vi "Start.vi"(8 "error in (no error)":errorcluster, 11 "SysLogbook in":refnum<class "SysLogbook.lvclass">) -> (0 "error out":errorcluster, 3 "SysLogbook out":refnum<class "SysLogbook.lvclass">)   [LabVIEW 2014, in "SysLogbook.lvclass"]
uses:
  SysLogbook.lvclass
  SysLogbook.lvclass/SysLogbook.ctl
  <vilib>/Utility/config.llb/Read Key (U32).vi
  <vilib>/Utility/config.llb/Read Key (Boolean).vi
  <vilib>/Utility/config.llb/Read Key (String).vi
  Logbook/Logbook.lvclass
  <vilib>/Utility/config.llb/NI_LVConfig.lvlib
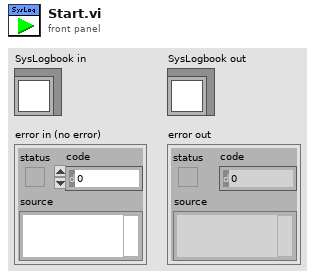
[diagram p1: front panel]
types:
  T1 = typedef "NI_LVConfig.lvlib/Config Data RefNum.ctl" = refnum<k1>
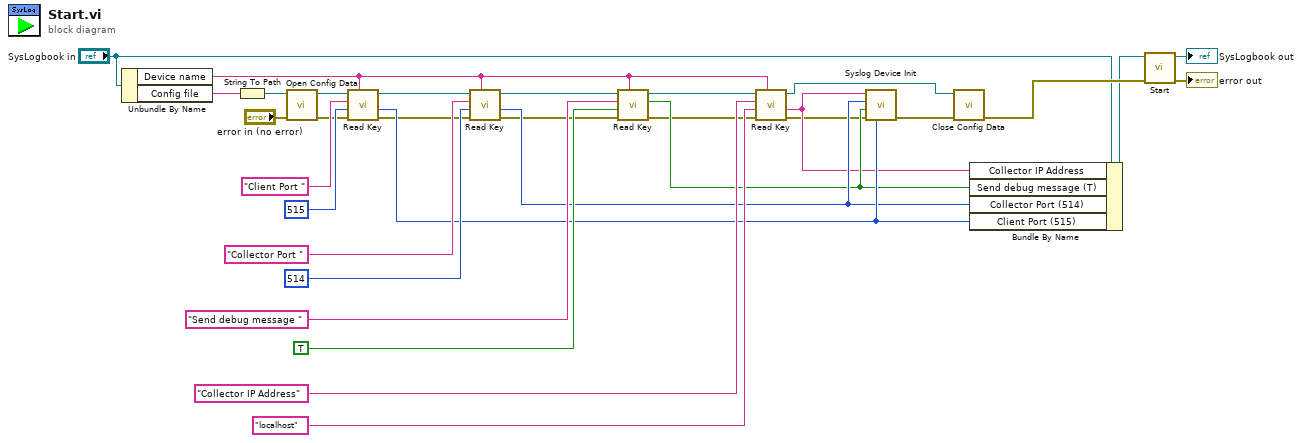
[diagram p0: block diagram]
diagram:
  n1 = Unbundle By Name("SysLogbook in") -> ("Device name"=w14:string, "Config file"=w16:string)
  n2 = String To Path(string=w16) -> (path=w15:path)
  n3 = call <vilib>:"Open Config Data.vi"("error in (no error)"="error in (no error)", "configuration file path"=w15) -> ("error out"=w3:errorcluster, "refnum"=w12:T1)  [unwired: 7 in, 1 out]
  n4 = call-poly <vilib>:"Read Key.vi"("section"=w14, "error in (no error)"=w3, "default value"=u16 515 ("Collector Port (514)"), "key"="Client Port ", "refnum"=w12) -> ("error out"=w4:errorcluster, "value"=w25:u32, "refnum out"=w11:T1)  [unwired: 3 in, 1 out]
  n5 = call-poly <vilib>:"Read Key.vi"("section"=w14, "error in (no error)"=w4, "default value"=u16 514 ("Client Port (515)"), "key"="Collector Port ", "refnum"=w11) -> ("error out"=w5:errorcluster, "value"=w24:u32, "refnum out"=w10:T1)  [unwired: 3 in, 1 out]
  n6 = call-poly <vilib>:"Read Key.vi"("section"=w14, "error in (no error)"=w5, "default value"=TRUE ("Send debug message (T)"), "key"="Send debug message ", "refnum"=w10) -> ("error out"=w6:errorcluster, "found?"=w23:bool, "refnum out"=w9:T1)  [unwired: 3 in, 1 out]
  n7 = call-poly <vilib>:"Read Key.vi"("section"=w14, "error in (no error)"=w6, "default value"="localhost" ("Collector IP Address"), "key"="Collector IP Address", "refnum"=w9) -> ("error out"=w2:errorcluster, "value"=w7:string, "refnum out"=w1:T1)  [unwired: 3 in, 1 out]
  n8 = call <vilib>:"Syslog Device Init.vi"("Client Port (515)"=w25, "error in (no error)"=w2, "Send debug message (T)"=w23, "Collector Port (514)"=w24, "Syslog Collector IP Address"=w7) -> ("error out"=w22:errorcluster)  [unwired: 6 in]
  n9 = call <vilib>:"Close Config Data.vi"("error in (no error)"=w22, "refnum"=w1) -> ("error out"=w26:errorcluster)  [unwired: 8 in, 1 out]
  n10 = Bundle By Name(cluster="SysLogbook in", "Collector IP Address"=w7, "Send debug message (T)"=w23, "Collector Port (514)"=w24, "Client Port (515)"=w25) -> (w17:refnum<class "SysLogbook.lvclass">)
  n11 = call-parent "Start.vi"("error in (no error)"=w26, "Logbook in"=w17) -> ("error out"=→"error out":errorcluster, "Logbook out"=→"SysLogbook out":refnum<class "SysLogbook.lvclass">)  [unwired: 8 in]
